vi "Centering.vi"() -> (3 "Ready To Move On":bool)   [LabVIEW 2011]
uses:
  Robot Global Data.vi
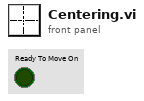
[diagram p1: front panel]
types:
  T1 = typedef "WPI_MotorControlDeviceRef.ctl" = cluster{"DeviceStatus":errorcluster, "Type":enum16{"PWM", "CAN"}, "PWM":cluster{"Digital Module":T2, "PWM Channel":T3, "DeadBand":T4}, "CAN":cluster{"Device Number":u8, "Control Mode":T5, "Semaphore":T6, "Max Vout":dbl}, "Invert":bool, "TransformRef":T7, "InvTransformRef":T7}
  T2 = typedef "FPGA_TypedefDigitalModule.ctl" = enum16{"Digital Module 1", "Digital Module 2"}
  T3 = typedef "FPGA_DIOPWMChannel.ctl" = enum8{"PWM 1", "PWM 2", "PWM 3", "PWM 4", "PWM 5", "PWM 6", "PWM 7", "PWM 8", "PWM 9", "PWM 10", "Invalid"}
  T4 = typedef "WPI_PWMDeadband.ctl" = cluster{"Name":string, "maxPositivePwm":i32, "minPositivePwm":i32, "centerPwm":i32, "maxNegativePwm":i32, "minNegativePwm":i32, "angularRange":u16}
  T5 = typedef "WPI_CANJaguar_ControlMode.ctl" = enum8{"Percent VBus", "Current", "Speed", "Position", "Voltage"}
  T6 = typedef "Semaphore RefNum" = refnum<k1>
  T7 = typedef "WPI_PWMTransform_ConPane.ctl" = refnum<vi>
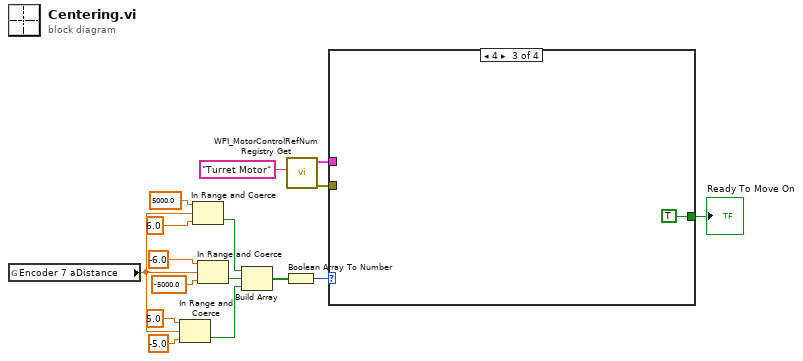
[diagram p0: block diagram]
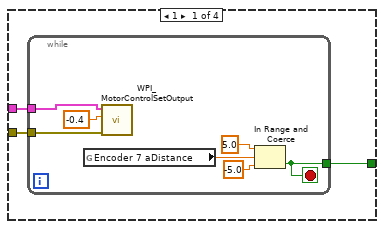
[diagram p2: hidden frame]
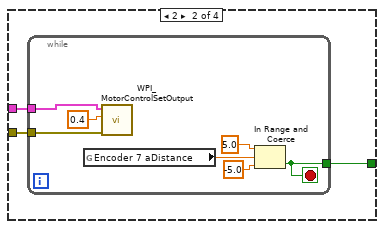
[diagram p3: hidden frame]
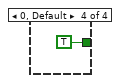
[diagram p4: hidden frame]
diagram:
  n1 = global read "Robot Global Data.vi" "Encoder 7 aDistance"() -> (w2:dbl)
  n2 = In Range and Coerce(upper limit=5.0, x=w2, lower limit=-5.0) -> (In Range?=w1:bool)  [unwired: 1 out]
  n3 = In Range and Coerce(upper limit=5000.0, x=w2, lower limit=6.0) -> (In Range?=w10:bool)  [unwired: 1 out]
  n4 = In Range and Coerce(upper limit=-6.0, x=w2, lower limit=-5000.0) -> (In Range?=w5:bool)  [unwired: 1 out]
  n5 = Build Array(w10, w5, w1) -> (w16:bool[])
  n6 = Boolean Array To Number(Boolean array=w16) -> (number=w15:u32)
  n7 = call <vilib>:"WPI_MotorControlRefNum Registry Get.vi"("refnum name"="Turret Motor") -> ("error out"=w12:errorcluster, "MotorControlDevRef"=w13:T1)  [unwired: 9 in]
  n8 = case shown="4" w15 {
    tunnel: w13 -> [w18 w29 _ _]
    tunnel: w12 -> [w17 w28 _ _]
    tunnel: [w19 w27 TRUE TRUE] -> w11
    frame 1 {
      n9 = while {
        tunnel: [w23] -> w19
        tunnel: w18 -> [w21]
        tunnel: w17 -> [w20]
        stop <- w23 stop-if-true
        n10 = global read "Robot Global Data.vi" "Encoder 7 aDistance"() -> (w26:dbl)
        n11 = call <vilib>:"WPI_MotorControlSetOutput.vi"("error in (no error)"=w20, "Output"=-0.4, "MotorControlDevRef"=w21) -> ()  [unwired: 7 in, 2 out]
        n12 = In Range and Coerce(upper limit=5.0, x=w26, lower limit=-5.0) -> (In Range?=w23:bool)  [unwired: 1 out]
      }
    }
    frame 2 {
      n13 = while {
        tunnel: [w34] -> w27
        tunnel: w29 -> [w32]
        tunnel: w28 -> [w31]
        stop <- w34 stop-if-true
        n14 = global read "Robot Global Data.vi" "Encoder 7 aDistance"() -> (w30:dbl)
        n15 = call <vilib>:"WPI_MotorControlSetOutput.vi"("error in (no error)"=w31, "Output"=0.4, "MotorControlDevRef"=w32) -> ()  [unwired: 7 in, 2 out]
        n16 = In Range and Coerce(upper limit=5.0, x=w30, lower limit=-5.0) -> (In Range?=w34:bool)  [unwired: 1 out]
      }
    }
    frame 4 {
    }
    frame 0, Default {
    }
  }
  "Ready To Move On" <- w11
